vi "Configure Reference And Phase.vi"(4 "Phase Mode (T: Auto Phase)":bool=TRUE, 5 "Reference Mode (T: Internal)":bool=TRUE, 6 "Phase (0.0)":dbl format="%.2e", 7 "Frequency (1.00E+6)":dbl=1000000.0 format="%.2e", 8 "Error In (no error)":errorcluster, 9 "Reference Input Impedance (0:50 ohm)":u16(ring) items=["50 ohm", "10 k ohm"], 10 "2F Mode (F: Off)":bool, 11 "VISA Resource Name":refnum<visa-resource-name>) -> (0 "Error Out":errorcluster, 3 "VISA Resource Name Out":refnum<visa-resource-name>)   [LabVIEW 2010, in "Stanford Research 844.lvlib"]
doc: "This VI configure reference and phase."
uses:
  <instrlib>/Stanford Research 844/Stanford Research 844.lvlib
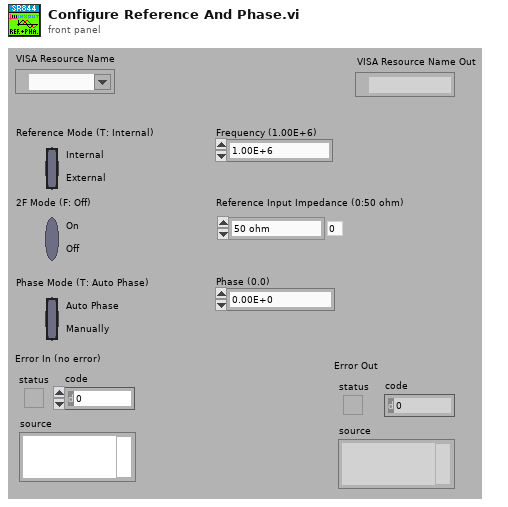
[diagram p1: front panel]
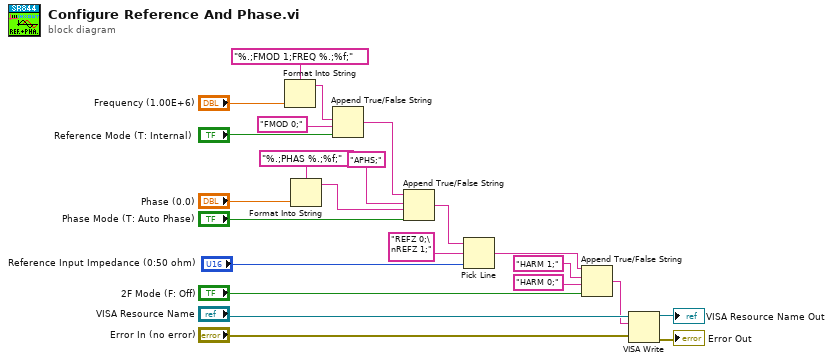
[diagram p0: block diagram]
diagram:
  n1 = Format Into String(format string="%.;FMOD 1;FREQ %.;%f;", "Frequency (1.00E+6)") -> (resulting string=w21:string)  [unwired: 2 in, 1 out]
  n2 = Format Into String(format string="%.;PHAS %.;%f;", "Phase (0.0)") -> (resulting string=w11:string)  [unwired: 2 in, 1 out]
  n3 = Append True/False String(1:"Reference Mode (T: Internal)", 2:"FMOD 0;" ("write buffer (\"\")"), 3:w21) -> (0:w6:string)  [unwired: 1 in]
  n4 = Append True/False String(1:"Phase Mode (T: Auto Phase)", 2:w11, 3:"APHS;" ("write buffer (\"\")"), 4:w6) -> (0:w3:string)
  n5 = Pick Line(string ("")=w3, multi-line string="REFZ 0;\nREFZ 1;", line index="Reference Input Impedance (0:50 ohm)") -> (output string=w4:string)
  n6 = Append True/False String(1:"2F Mode (F: Off)", 2:"HARM 0;" ("true string"), 3:"HARM 1;" ("true string"), 4:w4) -> (0:w5:string)
  n7 = VISA Write(VISA resource name="VISA Resource Name", write buffer=w5, error in (no error)="Error In (no error)") -> (VISA resource name out=→"VISA Resource Name Out":refnum<visa-resource-name>, error out=→"Error Out":errorcluster)  [unwired: 1 out]
